vi "Open File.vi"(7 "Access Mode (0: Read)":i32(ring) items=["Read"=0, "Write"=1, "Append"=2, "Nil"=4], 8 "error in (no error)":errorcluster, 9 "File Path":string, 10 "File Variable":string, 11 "VISA resource name":refnum<visa-resource-name>) -> (0 "error out":errorcluster, 3 "VISA resource name out":refnum<visa-resource-name>)   [LabVIEW 2015, in "Keithley 2600 Series.lvlib"]
doc: "Opens a file."
uses:
  Keithley 2600 Series.lvlib
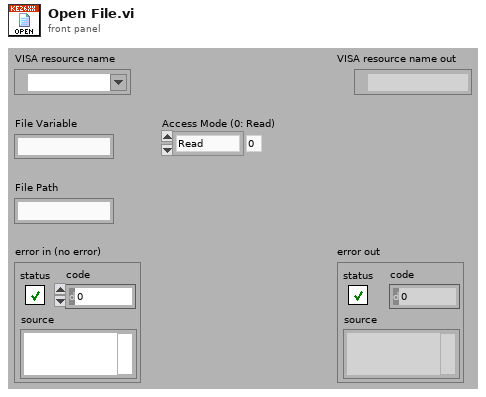
[diagram p1: front panel]
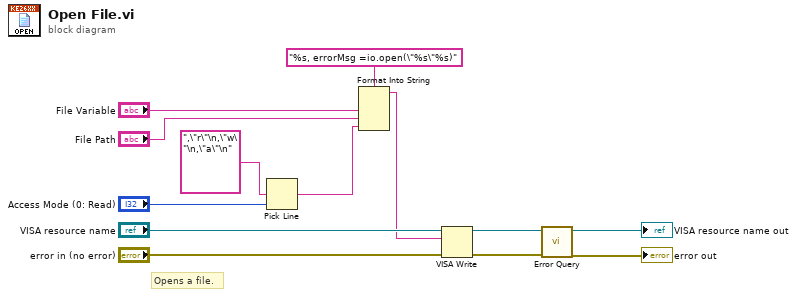
[diagram p0: block diagram]
diagram:
  # "Opens a file."
  n1 = Pick Line(multi-line string=",\"r\"\n,\"w\"\n,\"a\"\n", line index="Access Mode (0: Read)") -> (output string=w4:string)  [unwired: 1 in]
  n2 = Format Into String(format string="%s, errorMsg =io.open(\"%s\"%s)", "File Variable", "File Path", w4) -> (resulting string=w1:string)  [unwired: 2 in, 1 out]
  n3 = VISA Write(VISA resource name="VISA resource name", write buffer=w1, error in (no error)="error in (no error)") -> (VISA resource name out=w10:refnum<visa-resource-name>, error out=w9:errorcluster)  [unwired: 1 out]
  n4 = call "Error Query.vi"("error in (no error)"=w9, "VISA resource name"=w10) -> ("error out"=→"error out":errorcluster, "VISA resource name out"=→"VISA resource name out":refnum<visa-resource-name>)  [unwired: 6 in, 2 out]
